vi "AVS_PollScan.vi"(9 "a_hDevice":i32) -> (3 "Output Value":i32)   [LabVIEW 2013, in "Avantes Spectrometer Functions.lvlib"]
uses:
  Avantes Spectrometer Functions.lvlib
  AvantesSpectrometer2/polling_mc/AS5216.dll
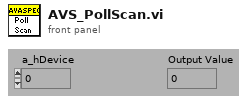
[diagram p1: front panel]
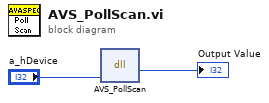
[diagram p0: block diagram]
diagram:
  n1 = dll-call lib="C:/Users/dhstuart/Dropbox/CLTC/AvantesSpectrometer2/polling_mc/AS5216.dll" fn="AVS_PollScan"("a_hDevice"="a_hDevice") -> (→"Output Value":i32)  [unwired: 4 in, 2 out]
